vi "NewMod.Tester.vi"() -> ()   [LabVIEW 2024]
uses:
  NewMod.lvclass/NewMod.ctl
  NewMod.lvclass
  JQMHCore/Module/RQMHModule.lvclass
  C:/DevOps/CORTEX/JQMH/JQMHCore/Module/RQMHModule.lvclass
  C:/DevOps/CORTEX/JQMH/ModuleTemplates/NewMod/NewMod.lvclass
panel:
  out "Last Error Time":timestamp
  out "last error":errorcluster
  out "Status":string
  in  "Tab Control":enum32{"Admin", "Commands"}(tab)
  in  "Stop Module":bool
  in  "Show Block Diagram":bool
  in  "Hide Module Panel":bool
  in  "Show Module Panel":bool
  in  "Start Module":bool
  in  "Hide Block Diagram":bool
  in  "Do Something":bool
  in  "Msg":string
  out "Value":dbl
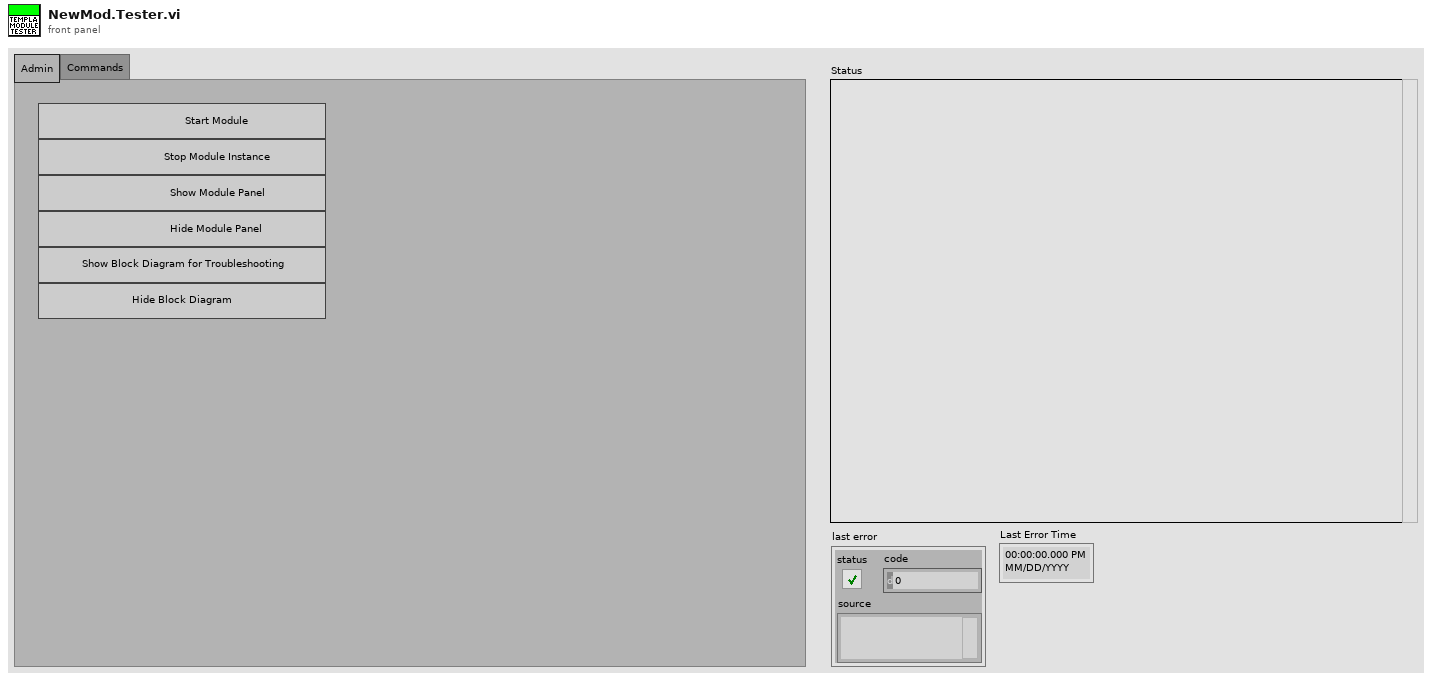
[diagram p1: front panel]
types:
  T1 = typedef "RQMHModule.lvclass/StandardBroadcasts.ctl" = cluster{"Died":refnum<user-event>, "Started":refnum<user-event>}
  T2 = typedef "NewMod.lvclass/Broadcast Events--cluster.ctl" = cluster{"Stopped":refnum<user-event>}
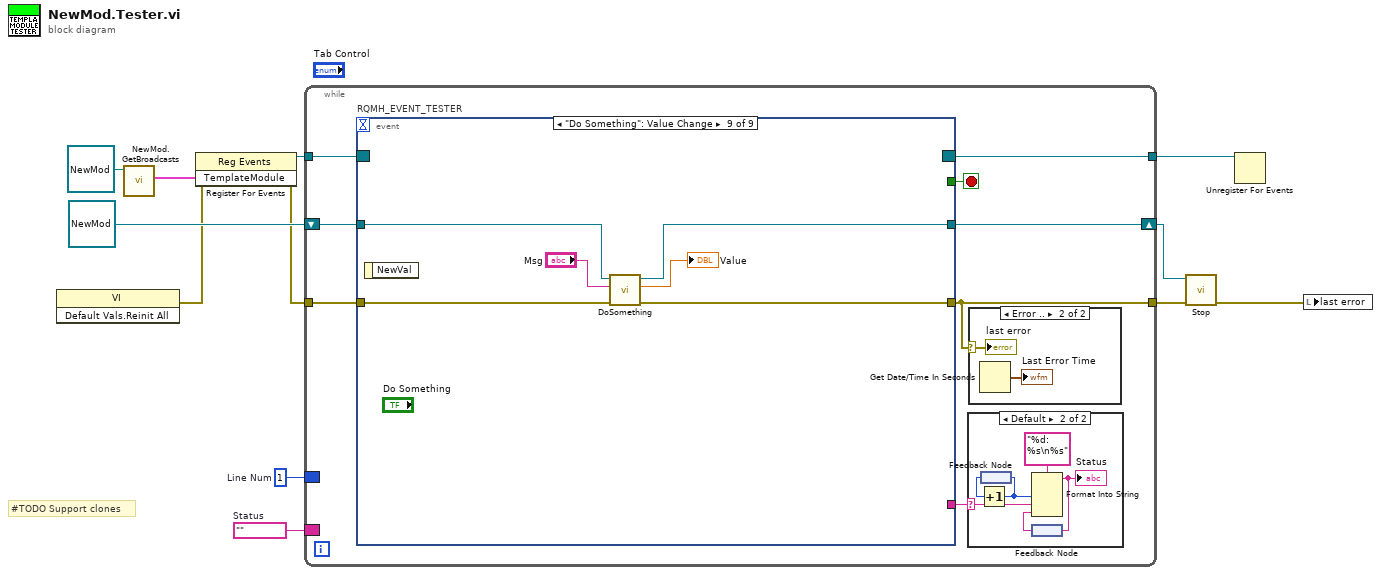
[diagram p0: block diagram]
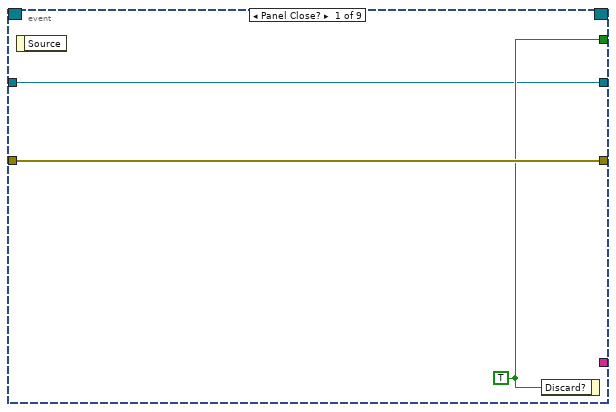
[diagram p2: hidden frame]
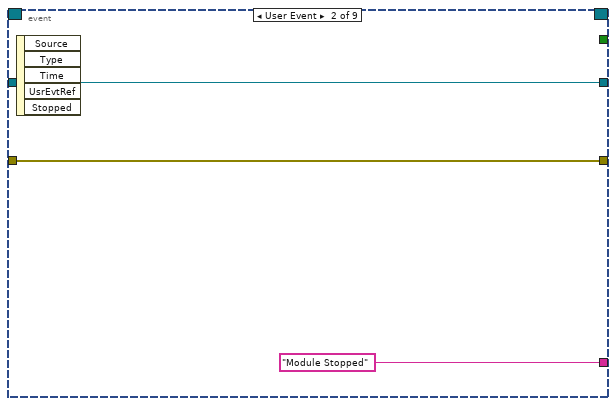
[diagram p3: hidden frame]
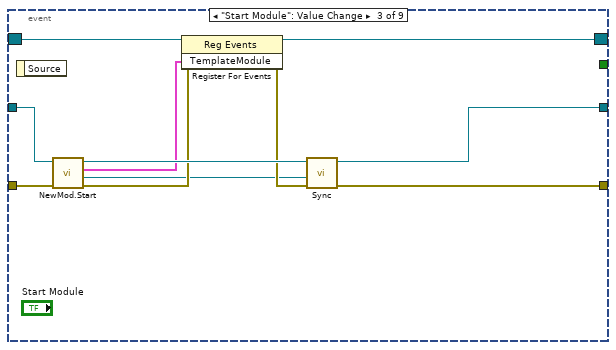
[diagram p4: hidden frame]
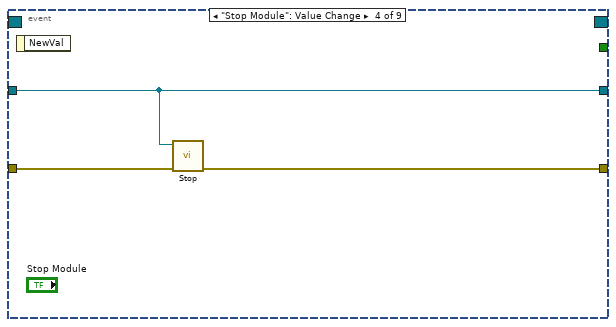
[diagram p5: hidden frame]
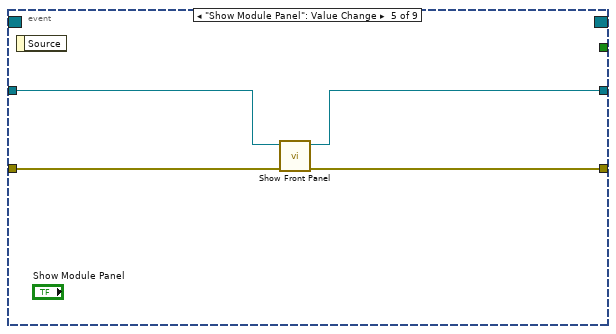
[diagram p6: hidden frame]
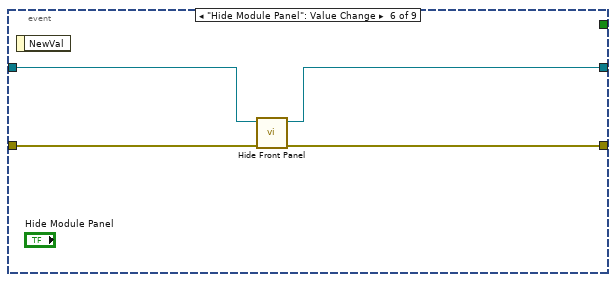
[diagram p7: hidden frame]
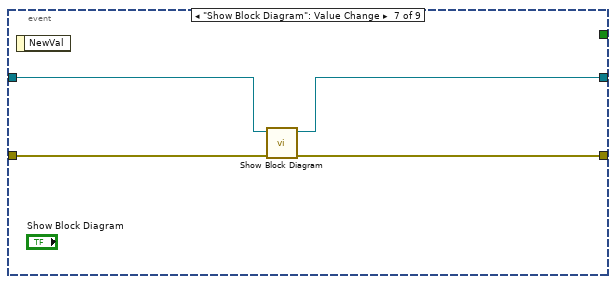
[diagram p8: hidden frame]
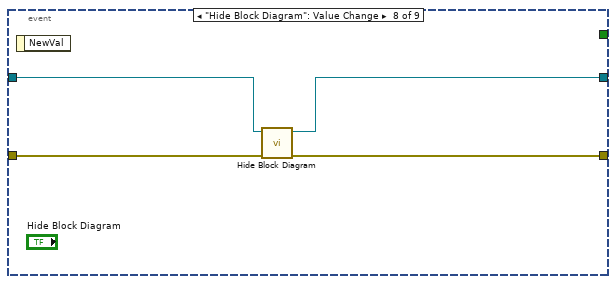
[diagram p9: hidden frame]
diagram:
  w1 = ""  # Status
  w2 = 1  # Line Num
  # "#TODO Support clones"
  n1 = invoke class="VI" method="Default Vals.Reinit All"() -> (error out=w7:errorcluster)  [unwired: 3 in, 2 out]
  n2 = call "NewMod.GetBroadcasts.vi"("NewTemplate in"=refnum<class "NewMod.lvclass"> refnum ("TemplateModule in")) -> ("TemplateModule"=w11:cluster{"Broadcasts":T1, "Broadcasts":T2})  [unwired: 9 in, 1 out]
  n3 = register-events(error in=w7, w11) -> (reference out=w10:refnum<event-registration>, error out=w6:errorcluster)  [unwired: 1 in]
  n4 = while {
    tunnel: w6 -> [w19]
    tunnel: w10 -> [w20]
    tunnel: [w18] -> w4
    tunnel: [w16] -> w9
    shift-right: [w14] -> w5
    shift-left: refnum<class "NewMod.lvclass"> refnum ("TemplateModule in") -> [w15]
    border: w2 -> [_]
    border: w1 -> [_]
    stop <- w17 stop-if-true
    n5 = event "RQMH_EVENT_TESTER" shown="[8] \"Do Something\": Value Change" {
      selector: w20 -> [_ _ w35 _ _ _ _ _ _]
      dyn-events: [_ _ w34 _ _ _ _ _ _] -> w16
      timeout: _ -> [_ _ _ _ _ _ _ _ _]
      tunnel: w19 -> [w23 w26 w37 w40 w43 w47 w51 w55 w61]
      tunnel: [w23 w26 w33 w39 w44 w48 w52 w53 w59] -> w18
      tunnel: [w22 _ _ _ _ _ _ _ _] -> w17
      tunnel: w15 -> [w21 w25 w36 w38 w41 w45 w49 w56 w62]
      tunnel: [w21 w25 w28 w38 w42 w46 w50 w54 w60] -> w14
      tunnel: [_ "Module Stopped" _ _ _ _ _ _ _] -> w13
      event Panel Close? {
        w22 = TRUE
        n6 = event-data() -> ()  [unwired: 1 in, 1 out]
        n7 = event-data("Discard?"=w22) -> ()  [unwired: 1 in, 1 out]
      }
      event User Event {
        n8 = event-data() -> ()  [unwired: 1 in, 5 out]
      }
      event "Start Module": Value Change {
        n9 = event-data() -> ()  [unwired: 1 in, 1 out]
        n10 = call "NewMod.Start.vi"("error in (no error)"=w37, "NewTemplate in"=w36) -> ("error out"=w31:errorcluster, "StartupHandshake out"=w29:refnum<class "RQMHStartup.lvclass">, "_TemplateModule"=w27:cluster{"Broadcasts":T1, "Broadcasts":T2}, "NewTemplate out"=w32:refnum<class "NewMod.lvclass">)  [unwired: 6 in]
        n11 = register-events(reference=w35, error in=w31, w27) -> (reference out=w34:refnum<event-registration>, error out=w30:errorcluster)
        n12 = call "Sync.vi"("error in (no error)"=w30, "StartupHandshake out"=w29, "JQMHCore in"=w32) -> ("error out"=w33:errorcluster, "JQMHCore out"=w28:refnum<class "NewMod.lvclass">)  [unwired: 7 in]
      }
      event "Stop Module": Value Change {
        n13 = event-data() -> ()  [unwired: 1 in, 1 out]
        n14 = call "Stop.vi"("error in (no error)"=w40, "JQMHCore in"=w38) -> ("error out"=w39:errorcluster)  [unwired: 9 in]
      }
      event "Show Module Panel": Value Change {
        n15 = event-data() -> ()  [unwired: 1 in, 1 out]
        n16 = call "Show Front Panel.vi"("error in (no error)"=w43, "JQMHCore in"=w41) -> ("error out"=w44:errorcluster, "JQMHCore out"=w42:refnum<class "NewMod.lvclass">)  [unwired: 8 in]
      }
      event "Hide Module Panel": Value Change {
        n17 = event-data() -> ()  [unwired: 1 in, 1 out]
        n18 = call "Hide Front Panel.vi"("error in (no error)"=w47, "JQMHCore in"=w45) -> ("error out"=w48:errorcluster, "JQMHCore out"=w46:refnum<class "NewMod.lvclass">)  [unwired: 8 in]
      }
      event "Show Block Diagram": Value Change {
        n19 = event-data() -> ()  [unwired: 1 in, 1 out]
        n20 = call "Show Block Diagram.vi"("error in (no error)"=w51, "JQMHCore in"=w49) -> ("error out"=w52:errorcluster, "JQMHCore out"=w50:refnum<class "NewMod.lvclass">)  [unwired: 8 in]
      }
      event "Hide Block Diagram": Value Change {
        n21 = event-data() -> ()  [unwired: 1 in, 1 out]
        n22 = call "Hide Block Diagram.vi"("error in (no error)"=w55, "JQMHCore in"=w56) -> ("error out"=w53:errorcluster, "JQMHCore out"=w54:refnum<class "NewMod.lvclass">)  [unwired: 8 in]
      }
      event "Do Something": Value Change {
        n23 = event-data() -> ()  [unwired: 1 in, 1 out]
        n24 = call "DoSomething.vi"("error in (no error)"=w61, "Msg"="Msg", "NewTemplate in"=w62) -> ("error out"=w59:errorcluster, "Value"=→"Value":dbl, "NewTemplate out"=w60:refnum<class "NewMod.lvclass">)  [unwired: 5 in, 1 out]
      }
    }
    n25 = case "RQMH_TESTER_STATUS" shown="Default" w13 {
      selector: w13 -> [_ w66]
      frame "" {
      }
      frame Default {
        n26 = feedback #1() -> (w65:i32)
        n27 = Increment(x=w65) -> (x+1=w64:i32)
        n28 = feedback-in #1(w64) -> ()
        n29 = feedback #2() -> (w67:string)
        n30 = Format Into String(format string="%d: %s\n%s", w64, w66, w67) -> (resulting string=w63:string)  [unwired: 2 in, 1 out]
        "Status" <- w63
        n31 = feedback-in #2(w63) -> ()
      }
    }
    n32 = case shown="Error .." w18 {
      selector: w18 -> [_ w70]
      frame No Error {
      }
      frame Error {
        n33 = Get Date/Time In Seconds() -> (seconds since 1Jan1904=→"Last Error Time":timestamp)
        "last error" <- w70
      }
    }
  }
  n34 = call "Stop.vi"("error in (no error)"=w4, "JQMHCore in"=w5) -> ("error out"=w3:errorcluster)  [unwired: 9 in]
  n35 = Unregister For Events(event registration refnum=w9) -> ()  [unwired: 1 in, 1 out]
  n36 = local write "last error"(w3) -> ()
